vi "system.GetPrivateEvents.vi"(8 "error in (no error)":errorcluster, 11 "lockin":refnum<class "system.lvclass">) -> (0 "error out":errorcluster, 2 "Private Events":T1, 3 "lockin out":refnum<class "system.lvclass">)   [LabVIEW 2019, in "system.lvclass"]
doc: "---------------------------------------------------------------\nJKI State Machine Objects™\nhttp://jki.net/state-machine-objects/\nCopyright (C) 2005-2015, JKI <info@jki.net>\nALL RIGHTS RESERVEDJKI State Machine Objects (SMO) 1.0.0.4\nJKI - JKI\nCopyright (c) 2015, JKI"
uses:
  system.lvclass
  Typedefs/PrivateEvents--lockin.output_config.ctl
  Typedefs/PrivateEvents--Cluster.ctl
  Typedefs/PrivateEvents--lockin.runCalculation.ctl
  Typedefs/PrivateEvents--lockin.lockin_REF_waveform.ctl
  DSP/Typedefs/LP_Config.ctl
  DSP/DSP.lvclass
  DSP.lockin/Typedefs/Lockin_Config.ctl
  DSP.lockin/DSP_lockin.lvclass
  <vilib>/Analysis/4window.llb/windowTd.ctl
  <vilib>/Analysis/NI_AALPro.lvlib
  <vilib>/measure/maspectr.llb/Power Spectrum and PSD Export Mode.ctl
  <vilib>/measure/NI_MAPro.lvlib
  DSP/Typedefs/FFT_Config.ctl
  Typedefs/PrivateEvents--system.Generator.configGenerator.ctl
  Generator/Typedefs/PrivateEvents--Generator.configGenerator.ctl
  Generator/Generator.lvclass
  Typedefs/PrivateEvents--system.DSP.runCalculation.ctl
  DSP/Typedefs/PrivateEvents--DSP.RunCalculation.ctl
  Typedefs/PrivateEvents--system.DAQ_Manager.setDAQConfig.ctl
  DAQmx.AO/Typedefs/AO.Terminal-enum.ctl
  DAQmx.AO/DAQmx.AO.lvclass
  DAQmx.AO/Typedefs/DAQmx.AO_Config.ctl
  DAQmx.AI/Typedefs/AI.Coupling-enum.ctl
  DAQmx.AI/DAQmx.AI.lvclass
  DAQmx.AI/Typedefs/AI.Terminal-enum.ctl
  DAQmx.AI/Typedefs/DAQmx.AI_Config.ctl
  DAQ_Manager/Typedefs/PrivateEvents--DAQ_Manager.setDAQConfig.ctl
  DAQ_Manager/DAQ_Manager.lvclass
panel:
  # "For instructions on how to use the JKI State Machine Objects, examples and video tutorials, visit:\nhttp://jki.net/state-machine-objects/\n\nJKI State Machine Objects™\nhttp://jki.net/state-machine-objects/\nCopyright (C) 2005-2015, JKI <info@jki.net>\nALL RIGHTS RESERVED"
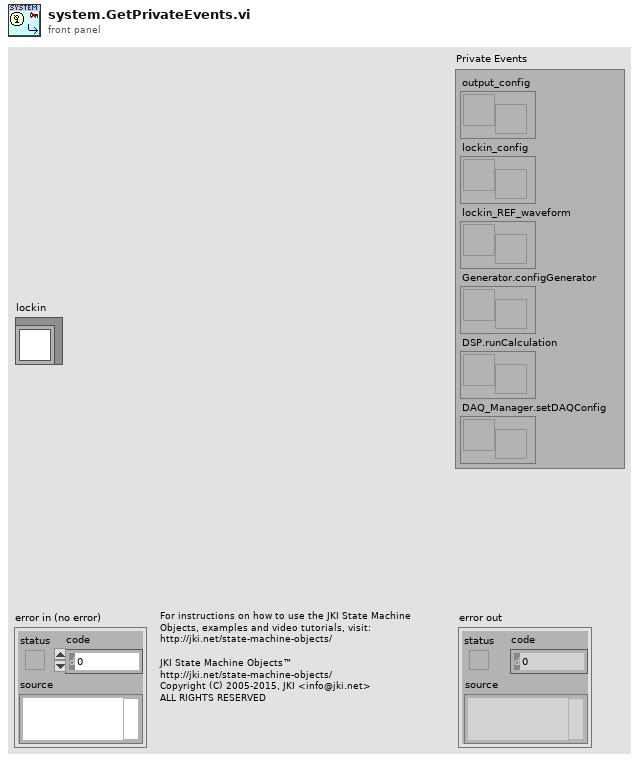
[diagram p1: front panel]
types:
  T1 = typedef "system.lvclass/PrivateEvents--Cluster.ctl" = cluster{"output_config":refnum<user-event>, "lockin_config":refnum<user-event>, "lockin_REF_waveform":refnum<user-event>, "Generator.configGenerator":refnum<user-event>, "DSP.runCalculation":refnum<user-event>, "DAQ_Manager.setDAQConfig":refnum<user-event>}
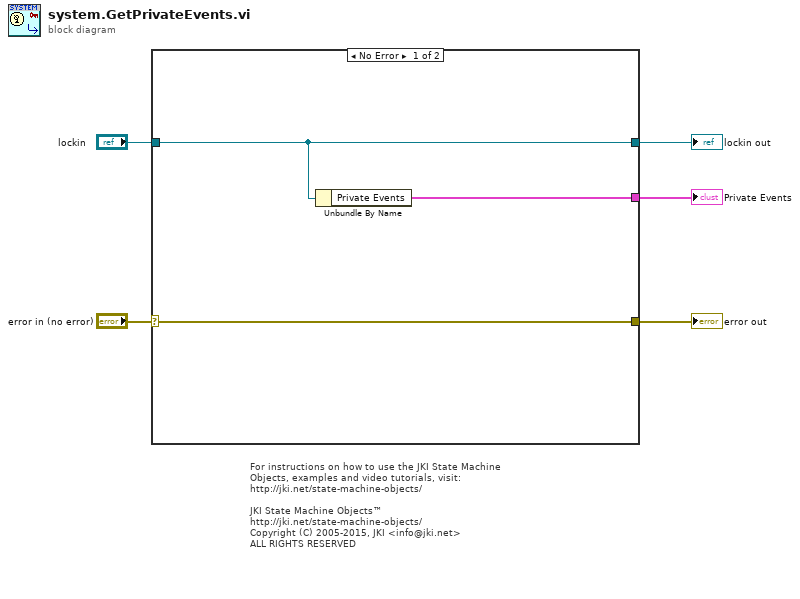
[diagram p0: block diagram]
diagram:
  # "For instructions on how to use the JKI State Machine Objects, examples and video tutorials, visit:\nhttp://jki.net/state-machine-objects/\n\nJKI State Machine Objects™\nhttp://jki.net/state-machine-objects/\nCopyright (C) 2005-2015, JKI <info@jki.net>\nALL RIGHTS RESERVED"
  n1 = case shown="No Error" "error in (no error)" {
    selector: "error in (no error)" -> [w7 w9]
    tunnel: "lockin" -> [w6 w10]
    tunnel: [w7 w9] -> w4
    tunnel: [w6 w10] -> w3
    tunnel: [w8 _] -> w1
    frame No Error {
      n2 = Unbundle By Name(w6) -> ("Private Events"=w8:T1)
    }
    frame Error {
    }
  }
  "error out" <- w4
  "lockin out" <- w3
  "Private Events" <- w1
